vi "ParseECHO.vi"(9 "指令返回的字符串":string) -> (2 "RX测量":string, 3 "TX测量":string)   [LabVIEW 2014]
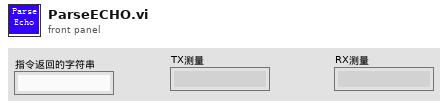
[diagram p1: front panel]
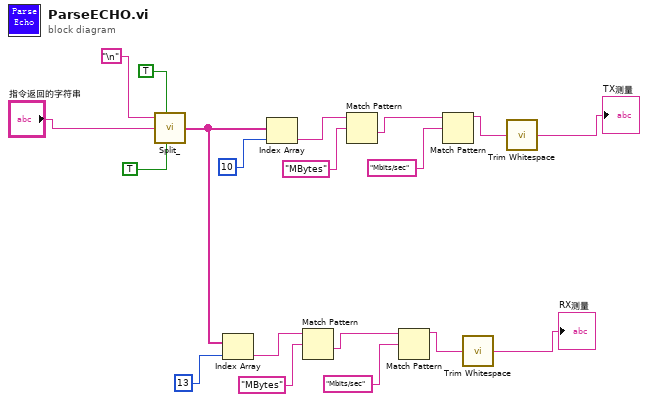
[diagram p0: block diagram]
diagram:
  n1 = call "Split_.vi"("分隔字符串/字符(,)"="\n", "移除空字符串（T）"=TRUE, "字符串"="指令返回的字符串", "移除空白字符（T）"=TRUE) -> ("字符串数组"=w1:string[])  [unwired: 3 in]
  n2 = Index Array(array=w1, index=13) -> (element=w6:string)
  n3 = Index Array(array=w1, index=10) -> (element=w13:string)
  n4 = Match Pattern(string=w6, regular expression="MBytes") -> (after substring=w5:string)  [unwired: 1 in, 3 out]
  n5 = Match Pattern(string=w13, regular expression="MBytes") -> (after substring=w12:string)  [unwired: 1 in, 3 out]
  n6 = Match Pattern(string=w5, regular expression="Mbits/sec") -> (before substring=w3:string)  [unwired: 1 in, 3 out]
  n7 = Match Pattern(string=w12, regular expression="Mbits/sec") -> (before substring=w10:string)  [unwired: 1 in, 3 out]
  n8 = call <vilib>:"Trim Whitespace.vi"("string"=w3) -> ("trimmed string"=→"RX测量":string)  [unwired: 1 in]
  n9 = call <vilib>:"Trim Whitespace.vi"("string"=w10) -> ("trimmed string"=→"TX测量":string)  [unwired: 1 in]
